vi "PE_MultipleAnalogAcquisition.vi"() -> ()   [LabVIEW 2016]
uses:
  <vilib>/Modbus/master/Create Master Instance (Serial).vi
  <vilib>/Modbus/master/Modbus Master.lvclass
  database/database.lvlib
panel:
  out "继电器":bool[](array[boolean])=[TRUE, TRUE, TRUE, TRUE, TRUE, TRUE, TRUE, TRUE]
  out "估算电阻":dbl[](array[numeric])
  in  "总压降":dbl=65535.0
  in  "参考电阻":dbl[](array[numeric])=[300.0, 300.0, 300.0, 300.0, 300.0, 300.0, 300.0, 300.0]
  out "JSON字符串":string
  in  "启动时间（毫秒）":u32=100
  in  "dataLabel":string
  in  "msg_id":dbl
  out "波形图表 2":dynamicdata(graph)
  in  "TestId":string
  out "AIn":u16[](array[numeric]) caption="测量值"
  # "Information Setting"
  # "Test Setting"
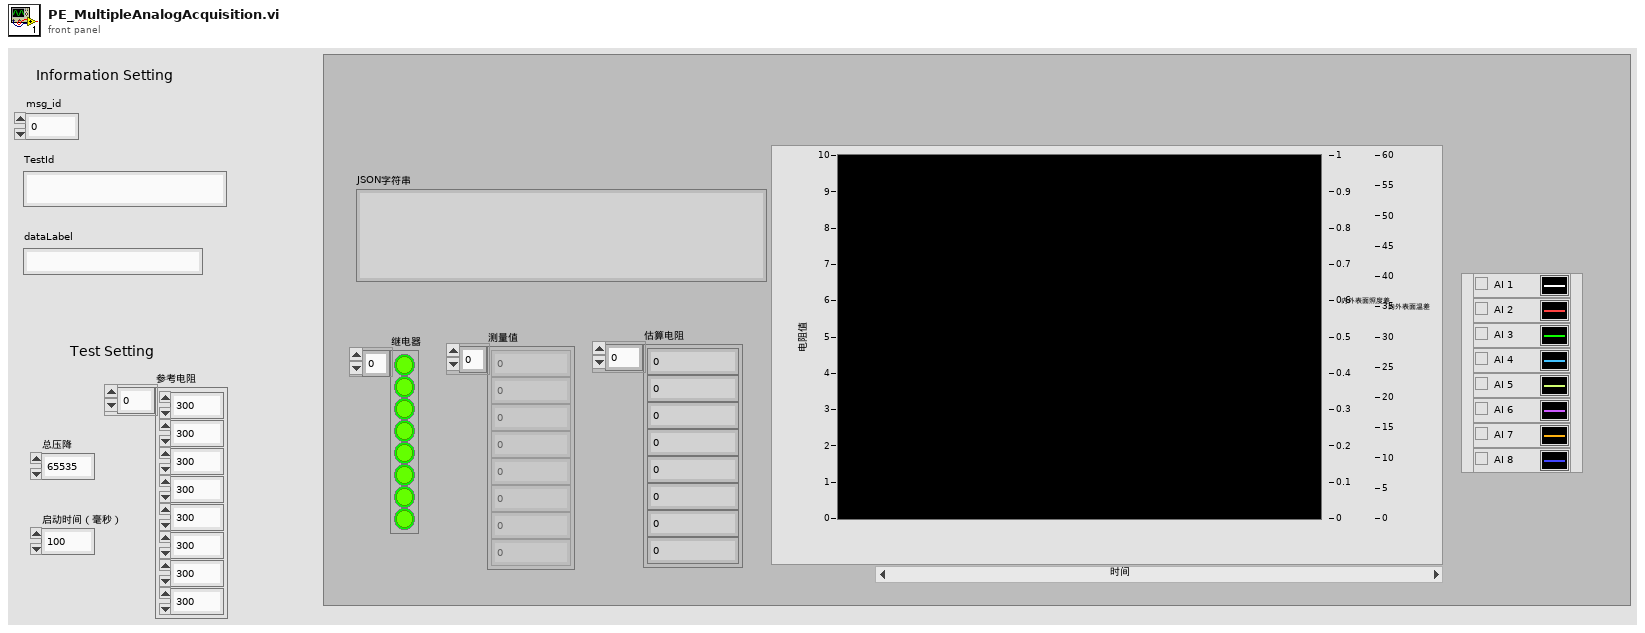
[diagram p1: front panel]
types:
  T1 = cluster{"AIn[0]":u16, "AIn[1]":u16, "AIn[2]":u16, "AIn[3]":u16, "AIn[4]":u16, "AIn[5]":u16, "AIn[6]":u16, "AIn[7]":u16, "AIn[8]":u16}
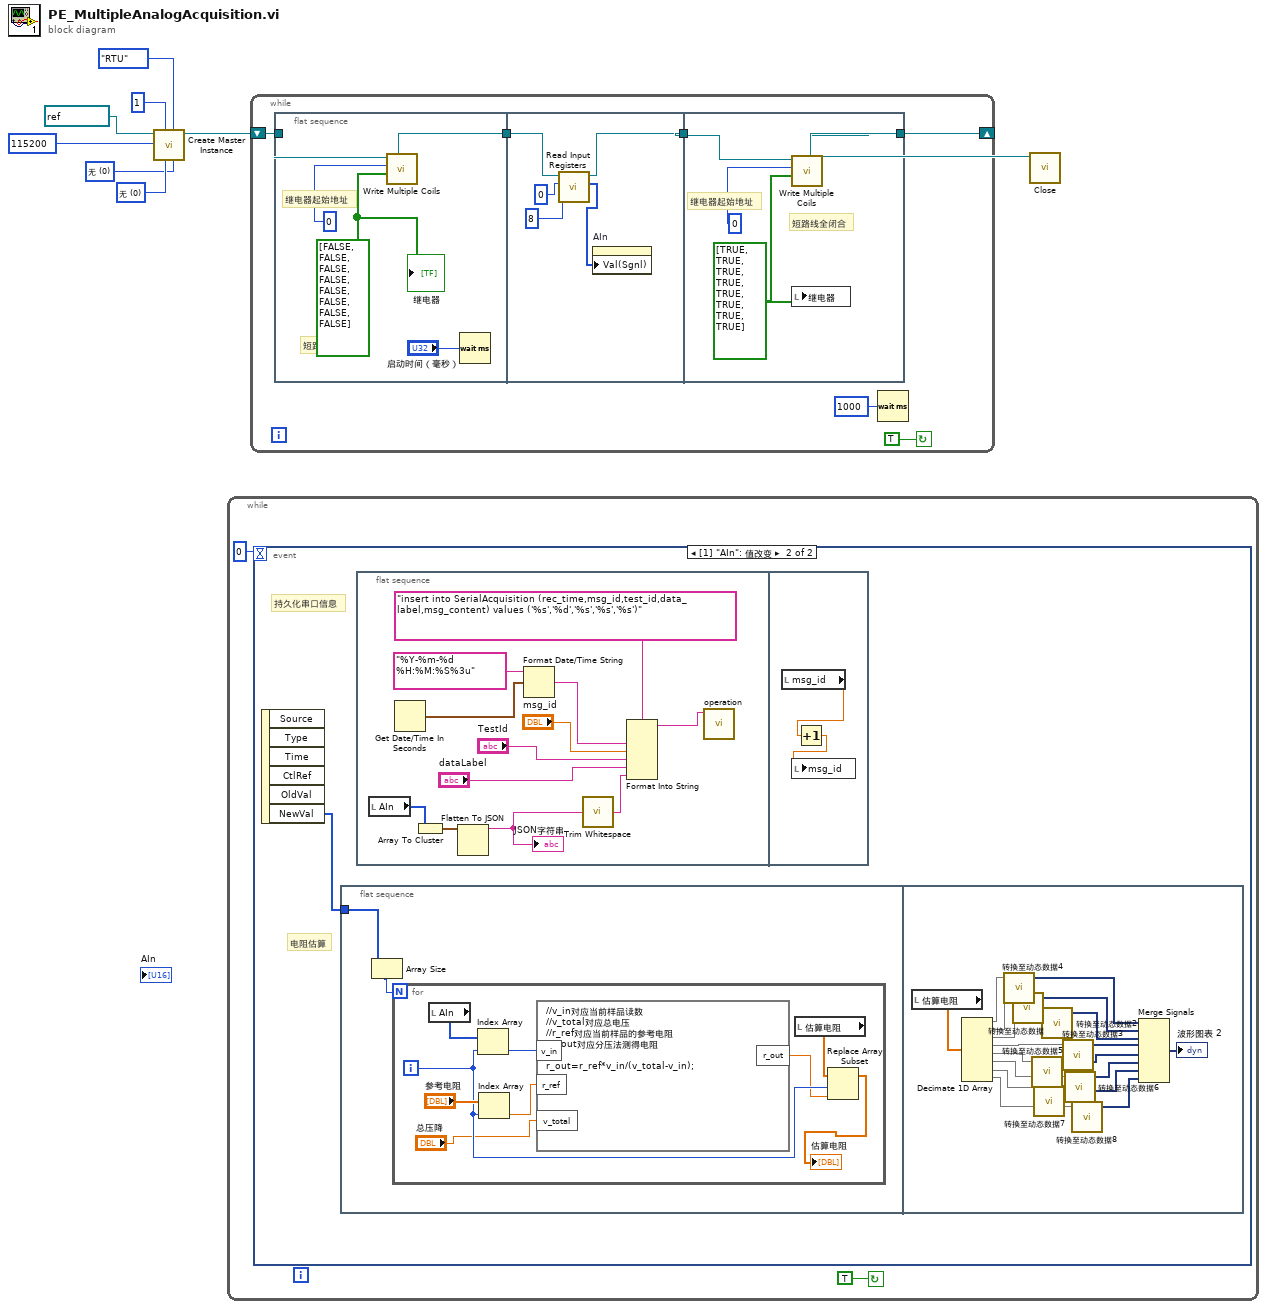
[diagram p0: block diagram]
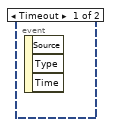
[diagram p2: hidden frame]
diagram:
  w3 = u16 0 items=["无", "XON/XOFF", "RTS/CTS", "XON/XOFF & RTS/CTS", "DTR/DSR", "XON/XOFF & DTR/DSR"] ("flow control (None)")
  w4 = u16 0 items=["无", "奇", "偶"] ("parity (Even)")
  n1 = call-poly <vilib>:"Create Master Instance.vi"("flow control (None)"=w3, "serial type"=enum16{"RTU", "ASCII"}."RTU", "parity (Even)"=w4, "unit ID"=u8 1, "baud rate (9600)"=u32 115200, "VISA resource name"=refnum<visa-resource-name> "COM5") -> ("serial master instance"=w2:refnum<class "Modbus Master.lvclass">)  [unwired: 4 in, 1 out]
  n2 = while {
    stop <- TRUE continue-if-true
    n3 = event shown="[1] \"AIn\": 值改变" {
      selector: _ -> [_ _]
      dyn-events: _ -> [_ _]
      timeout: 0 -> [_ _]
      event Timeout {
        n4 = event-data() -> ()  [unwired: 1 in, 3 out]
      }
      event "AIn": Value Change {
        # "电阻估算"
        # "持久化串口信息"
        n5 = event-data() -> ("NewVal"=w11:u16[])  [unwired: 1 in, 5 out]
        n6 = flat-sequence {
          tunnel: w11 -> [w12]
          frame #0 {
            n7 = Array Size(array=w12) -> (size(s)=w13:i32)
            n8 = for {
              N: w13 -> [_]
              i -> [w18]
              n9 = local read "AIn"() -> (w15:u16[])
              n10 = Index Array(array=w15, index=w18) -> (element=w20:u16)
              n11 = Index Array(array="参考电阻", index=w18) -> (element=w21:dbl)
              n12 = formula code="//v_in对应当前样品读数\n//v_total对应总电压\n//r_ref对应当前样品的参考电阻\n//r_out对应分压法测得电阻\n\nr_out=r_ref*v_in/(v_total-v_in);"("v_in"=w20, "r_ref"=w21, "v_total"="总压降") -> ("r_out"=w17:dbl)
              n13 = local read "估算电阻"() -> (w19:dbl[])
              n14 = Replace Array Subset(array=w19, new element=w17, index=w18) -> (→"估算电阻":dbl[])
            }
          }
          frame #1 {
            n15 = local read "估算电阻"() -> (w40:dbl[])
            n16 = Decimate 1D Array(w40) -> (w39:dbl[], w37:dbl[], w35:dbl[], w33:dbl[], w31:dbl[], w29:dbl[], w27:dbl[], w25:dbl[])
            n17 = call "转换至动态数据4"("Array"=w39) -> ("Dynamic Data Type"=w38:dynamicdata)  [unwired: 3 in]
            n18 = call "转换至动态数据"("Array"=w37) -> ("Dynamic Data Type"=w36:dynamicdata)  [unwired: 3 in]
            n19 = call "转换至动态数据5"("Array"=w31) -> ("Dynamic Data Type"=w30:dynamicdata)  [unwired: 3 in]
            n20 = call "转换至动态数据7"("Array"=w27) -> ("Dynamic Data Type"=w26:dynamicdata)  [unwired: 3 in]
            n21 = call "转换至动态数据2"("Array"=w35) -> ("Dynamic Data Type"=w34:dynamicdata)  [unwired: 3 in]
            n22 = call "转换至动态数据3"("Array"=w33) -> ("Dynamic Data Type"=w32:dynamicdata)  [unwired: 3 in]
            n23 = call "转换至动态数据6"("Array"=w29) -> ("Dynamic Data Type"=w28:dynamicdata)  [unwired: 3 in]
            n24 = call "转换至动态数据8"("Array"=w25) -> ("Dynamic Data Type"=w24:dynamicdata)  [unwired: 3 in]
            n25 = Merge Signals(w38, w36, w34, w32, w30, w28, w26, w24) -> (→"波形图表 2":dynamicdata)
          }
        }
        n26 = flat-sequence {
          frame #0 {
            n27 = local read "AIn"() -> (w42:u16[])
            n28 = Get Date/Time In Seconds() -> (seconds since 1Jan1904=w50:timestamp)
            n29 = Array To Cluster(array=w42) -> (cluster=w45:T1)
            n30 = Flatten To JSON(anything=w45) -> (JSON string=w44:string)  [unwired: 2 in, 1 out]
            "JSON字符串" <- w44
            n31 = Format Date/Time String ("格式化日期/时间字符串")(time format string (%c)="%Y-%m-%d %H:%M:%S%3u" ("时间格式字符串(%c)"), seconds (now)=w50) -> (date/time string=w48:string)  [unwired: 1 in]
            n32 = call <vilib>:"Trim Whitespace.vi"("string"=w44) -> ("trimmed string"=w49:string)  [unwired: 1 in]
            n33 = Format Into String(format string="insert into SerialAcquisition (rec_time,msg_id,test_id,data_label,msg_content) values ('%s','%d','%s','%s','%s')" ("格式字符串"), w48, "msg_id", "TestId", "dataLabel", w49) -> (resulting string=w43:string)  [unwired: 2 in, 1 out]
            n34 = call "operation.vi"("Command Text"=w43) -> ()  [unwired: 9 in, 1 out]
          }
          frame #1 {
            n35 = local read "msg_id"() -> (w54:dbl)
            n36 = Increment(x=w54) -> (x+1=w53:dbl)
            n37 = local write "msg_id"(w53) -> ()
          }
        }
      }
    }
  }
  n38 = while {
    shift-right: [w59] -> w1
    shift-left: w2 -> [w60]
    stop <- TRUE continue-if-true
    n39 = flat-sequence {
      tunnel: w60 -> [w65]
      tunnel: [w64] -> w57
      tunnel: w57 -> [w68]
      tunnel: [w67] -> w56
      tunnel: [w72] -> w59
      tunnel: w56 -> [w73]
      frame #0 {
        w61 = bool[] [FALSE, FALSE, FALSE, FALSE, FALSE, FALSE, FALSE, FALSE] ("coil values")
        # "短路口全断开"
        # "继电器起始地址"
        n40 = call-dynamic "Write Multiple Coils.vi"("coil values"=w61, "starting address"=u16 0, "Modbus master in"=w65) -> ("Modbus master out"=w64:refnum<class "Modbus Master.lvclass">)  [unwired: 7 in, 1 out]
        n41 = Wait (ms)(milliseconds to wait="启动时间（毫秒）") -> ()  [unwired: 1 out]
        "继电器" <- w61
      }
      frame #1 {
        n42 = call-dynamic "Read Input Registers.vi"("number of input registers"=u16 8 ("number of holding registers"), "starting address"=u16 0, "Modbus master in"=w68) -> ("register values"=w66:u16[], "Modbus master out"=w67:refnum<class "Modbus Master.lvclass">)  [unwired: 6 in, 1 out]
        n43 = property on="AIn" class="Arr (严格)"("Val(Sgnl)"=w66) -> ()  [unwired: 2 in, 2 out]
      }
      frame #2 {
        w71 = bool[] [TRUE, TRUE, TRUE, TRUE, TRUE, TRUE, TRUE, TRUE] ("coil values")
        # "短路线全闭合"
        # "继电器起始地址"
        n44 = call-dynamic "Write Multiple Coils.vi"("coil values"=w71, "starting address"=u16 0, "Modbus master in"=w73) -> ("Modbus master out"=w72:refnum<class "Modbus Master.lvclass">)  [unwired: 7 in, 1 out]
        n45 = local write "继电器"(w71) -> ()
      }
    }
    n46 = Wait (ms)(milliseconds to wait=u32 1000 ("等待时间（毫秒）")) -> ()  [unwired: 1 out]
  }
  n47 = call-dynamic "Close.vi"("Modbus master in"=w1) -> ()  [unwired: 10 in, 1 out]
